vi "Make filepath.vi"(8 "error in (no error)":errorcluster, 9 "is cxd file path?":bool, 10 "base path":path, 11 "DAQOrcaFlash in":refnum<class "DAQOrcaFlash.lvclass">) -> (0 "error out":errorcluster, 2 "filepath out":path, 3 "DAQOrcaFlash out":refnum<class "DAQOrcaFlash.lvclass">)   [LabVIEW 2012, in "DAQOrcaFlash.lvclass"]
uses:
  DAQOrcaFlash.lvclass
  DAQOrcaFlash.lvclass/DAQOrcaFlash.ctl
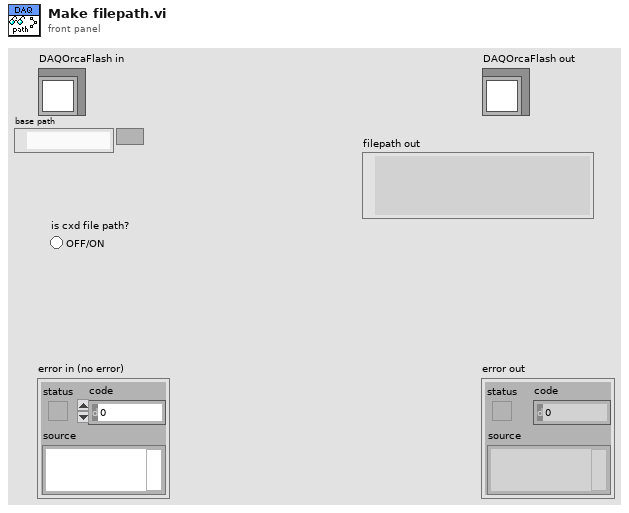
[diagram p1: front panel]
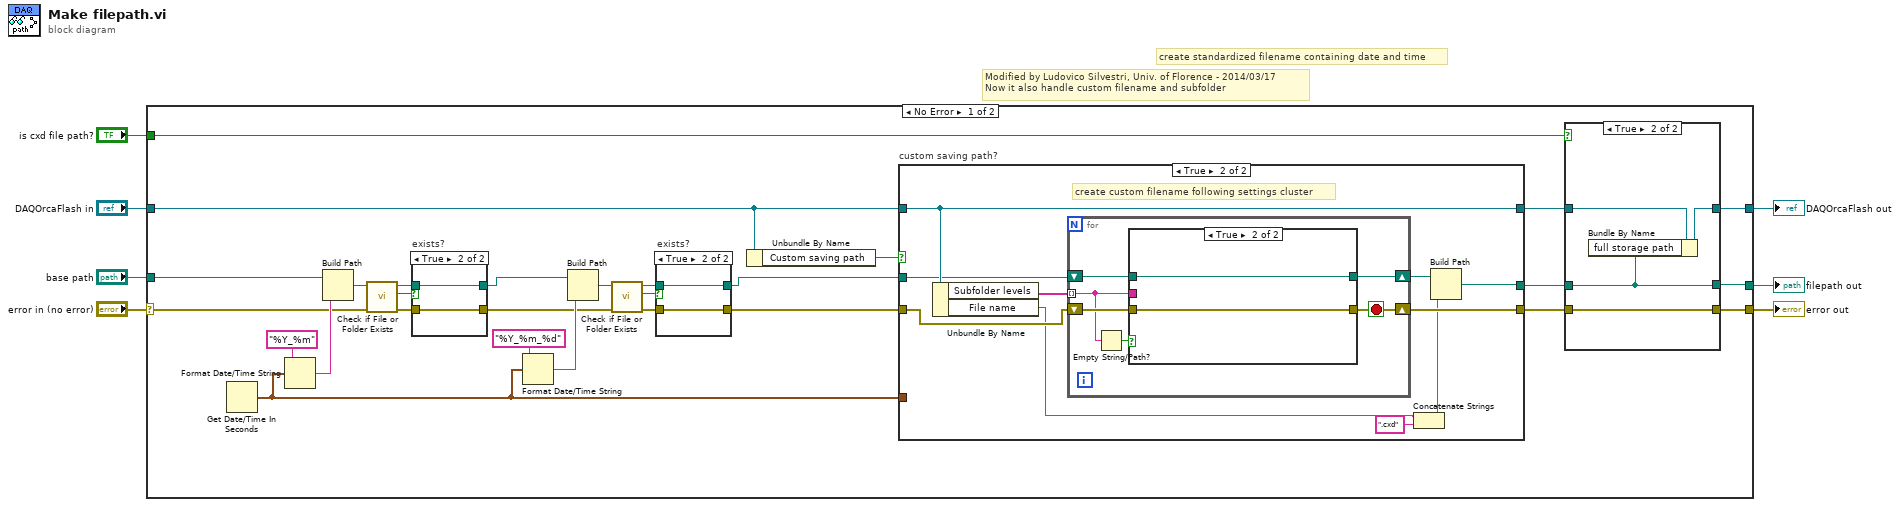
[diagram p0: block diagram]
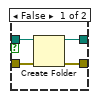
[diagram p3: hidden frame]
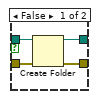
[diagram p4: hidden frame]
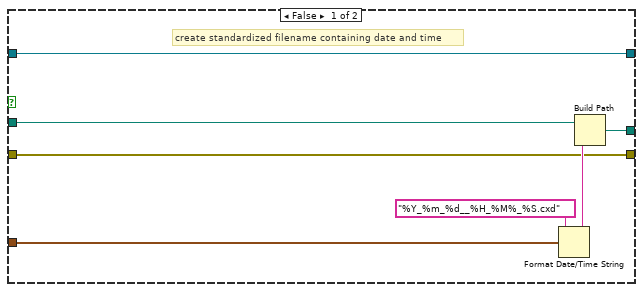
[diagram p5: hidden frame]
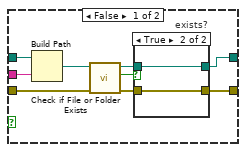
[diagram p6: hidden frame]
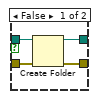
[diagram p7: hidden frame]
diagram:
  # "create standardized filename containing date and time"
  # "Modified by Ludovico Silvestri, Univ. of Florence - 2014/03/17\nNow it also handle custom filename and subfolder"
  n1 = case shown="No Error" "error in (no error)" {
    selector: "error in (no error)" -> [w20 w96]
    tunnel: [w9 w96] -> w6
    tunnel: [w13 w95] -> w5
    tunnel: "DAQOrcaFlash in" -> [w19 w95]
    tunnel: [w11 _] -> w4
    tunnel: "base path" -> [w15 _]
    tunnel: "is cxd file path?" -> [w8 _]
    frame No Error {
      n2 = Get Date/Time In Seconds() -> (seconds since 1Jan1904=w17:timestamp)
      n3 = Format Date/Time String(time format string (%c)="%Y_%m", seconds (now)=w17) -> (date/time string=w34:string)  [unwired: 1 in]
      n4 = Build Path(base path=w15, name or relative path=w34) -> (appended path=w32:path)
      n5 = call <vilib>:"Check if File or Folder Exists.vi"("error in (no error)"=w20, "path"=w32) -> ("error out"=w29:errorcluster, "file or folder exists?"=w31:bool, "dup path"=w30:path)  [unwired: 7 in]
      n6 = case "exists?" shown="True" w31 {
        tunnel: w30 -> [w51 w53]
        tunnel: w29 -> [w52 w54]
        tunnel: [w50 w53] -> w21
        tunnel: [w49 w54] -> w22
        frame False {
          n7 = Create Folder(path (use dialog)=w51, error in=w52) -> (created path=w50:path, error out=w49:errorcluster)  [unwired: 1 in, 1 out]
        }
        frame True {
        }
      }
      n8 = Format Date/Time String(time format string (%c)="%Y_%m_%d", seconds (now)=w17) -> (date/time string=w24:string)  [unwired: 1 in]
      n9 = Build Path(base path=w21, name or relative path=w24) -> (appended path=w28:path)
      n10 = call <vilib>:"Check if File or Folder Exists.vi"("error in (no error)"=w22, "path"=w28) -> ("error out"=w25:errorcluster, "file or folder exists?"=w27:bool, "dup path"=w26:path)  [unwired: 7 in]
      n11 = case "exists?" shown="True" w27 {
        tunnel: w26 -> [w45 w47]
        tunnel: w25 -> [w46 w48]
        tunnel: [w44 w47] -> w16
        tunnel: [w43 w48] -> w18
        frame False {
          n12 = Create Folder(path (use dialog)=w45, error in=w46) -> (created path=w44:path, error out=w43:errorcluster)  [unwired: 1 in, 1 out]
        }
        frame True {
        }
      }
      n13 = Unbundle By Name(w19) -> ("Custom saving path"=w35:bool)
      n14 = case "custom saving path?" shown="True" w35 {
        tunnel: w18 -> [w57 w66]
        tunnel: w19 -> [w60 w71]
        tunnel: [w57 w67] -> w10
        tunnel: [w59 w68] -> w12
        tunnel: [w60 w71] -> w14
        tunnel: w17 -> [w55 _]
        tunnel: w16 -> [w56 w62]
        frame False {
          # "create standardized filename containing date and time"
          n15 = Format Date/Time String(time format string (%c)="%Y_%m_%d__%H_%M%_%S.cxd", seconds (now)=w55) -> (date/time string=w61:string)  [unwired: 1 in]
          n16 = Build Path(base path=w56, name or relative path=w61) -> (appended path=w59:path)
        }
        frame True {
          # "create custom filename following settings cluster"
          n17 = Unbundle By Name(w71) -> ("Subfolder levels"=w70:string[], "File name"=w65:string)
          n18 = for {
            tunnel: w70 -> [w73] mode=indexing
            shift-right: [w75] -> w69
            shift-left: w62 -> [w77]
            shift-right: [w74] -> w67
            shift-left: w66 -> [w76]
            stop <- w74 stop-if-true
            n19 = Empty String/Path?(string/path=w73) -> (empty?=w72:bool)
            n20 = case shown="True" w72 {
              tunnel: w77 -> [w86 w93]
              tunnel: w73 -> [w85 _]
              tunnel: w76 -> [w80 w94]
              tunnel: [w79 w93] -> w75
              tunnel: [w78 w94] -> w74
              frame False {
                n21 = Build Path(base path=w86, name or relative path=w85) -> (appended path=w81:path)
                n22 = call <vilib>:"Check if File or Folder Exists.vi"("error in (no error)"=w80, "path"=w81) -> ("error out"=w84:errorcluster, "file or folder exists?"=w82:bool, "dup path"=w83:path)  [unwired: 7 in]
                n23 = case "exists?" shown="True" w82 {
                  tunnel: w83 -> [w89 w91]
                  tunnel: w84 -> [w90 w92]
                  tunnel: [w88 w91] -> w79
                  tunnel: [w87 w92] -> w78
                  frame False {
                    n24 = Create Folder(path (use dialog)=w89, error in=w90) -> (created path=w88:path, error out=w87:errorcluster)  [unwired: 1 in, 1 out]
                  }
                  frame True {
                  }
                }
              }
              frame True {
              }
            }
          }
          n25 = Concatenate Strings(w65, ".cxd" ("string")) -> (w63:string)
          n26 = Build Path(base path=w69, name or relative path=w63) -> (appended path=w68:path)
        }
      }
      n27 = case shown="True" w8 {
        tunnel: w14 -> [w38 w42]
        tunnel: [w38 w41] -> w13
        tunnel: w12 -> [w37 w40]
        tunnel: [w37 w40] -> w11
        tunnel: w10 -> [w36 w39]
        tunnel: [w36 w39] -> w9
        frame False {
        }
        frame True {
          n28 = Bundle By Name(cluster=w42, "full storage path"=w40) -> (w41:refnum<class "DAQOrcaFlash.lvclass">)
        }
      }
    }
    frame Error {
    }
  }
  "error out" <- w6
  "DAQOrcaFlash out" <- w5
  "filepath out" <- w4
